vi "ConvertPB_LongDelay.vi"(0 "PB VLIW Array in":T2(array[cluster]) {"Output Bits" format="%x"}, 1 "Definitions":T1={"External MemorySize"=32768, "Internal Memory Size"=512, "Overhead Ticks"=3, "Min Delay Loops"=3, "Loop Count Correction"=1, "Long Delay Loop Count Correction"=2, "Min Instruction Ticks"=6, "Long Delay Ticks"=4294967295, "Clock Period (s)"=1e-08, "Overhead Time (s)"=3e-08, "Min Instruction Cycle Time (s)"=9e-08, "Long Delay Time (s) "=42.94967298} {"Long Delay Time (s)" format="%.8p"; "Min Instruction Cycle Time (s)" format="%.0p"; "Overhead Time (s)" format="%.0p"; "Clock Period (s)" format="%.0p"; "Long Delay Ticks" format="%.0x"}, 2 "error in (no error)":errorcluster, 3 "Full trigger mask":u32 format="%x") -> (5 "PB VLIW Array out":T2(array[cluster]) {"Output Bits" format="%x"}, 6 "error out":errorcluster)   [LabVIEW 2013, in "PulseBlaster.lvlib"]
doc: "Accounts for the strange clocking in of the line following a trigger while the PB is waiting for an external analog trigger."
uses:
  PulseBlaster.lvlib
panel:
  in  "BeginLoop pointer":u32
  # "(Period*Long D Ticks)+Overhead time"
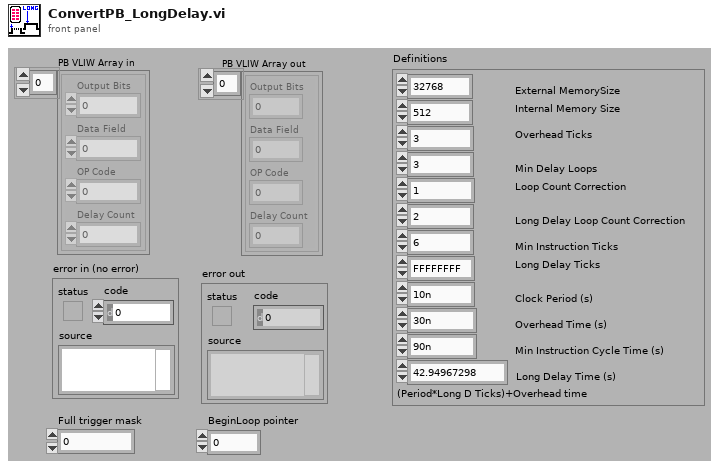
[diagram p1: front panel]
types:
  T1 = cluster{"External MemorySize":u16, "Internal Memory Size":u16, "Overhead Ticks":u8, "Min Delay Loops":u8, "Loop Count Correction":u8, "Long Delay Loop Count Correction":u8, "Min Instruction Ticks":u8, "Long Delay Ticks":u64, "Clock Period (s)":dbl, "Overhead Time (s)":dbl, "Min Instruction Cycle Time (s)":dbl, "Long Delay Time (s) ":dbl}
  T2 = cluster{"Output Bits":u32, "Data Field":u32, "OP Code":u8, "Delay Count":u64}[]
  T3 = cluster{"Output Bits":u32, "Data Field":u32, "OP Code":u8, "Delay Count":u32}[]
  T4 = cluster{"Output Bits":u32, "Data Field":u32, "OP Code":u8, u32}
  T5 = cluster{"Output Bits":u32, "Data Field":u32, "OP Code":u8, "Delay Count":u64}
  T6 = cluster{"Output Bits":u32, "BeginLoop pointer":u32, "OP Code":u8, "Delay Count":u64}
  T7 = cluster{"Output Bits":u32, "BeginLoop pointer":u32, "OP Code":u8, "Delay Count":u64}[]
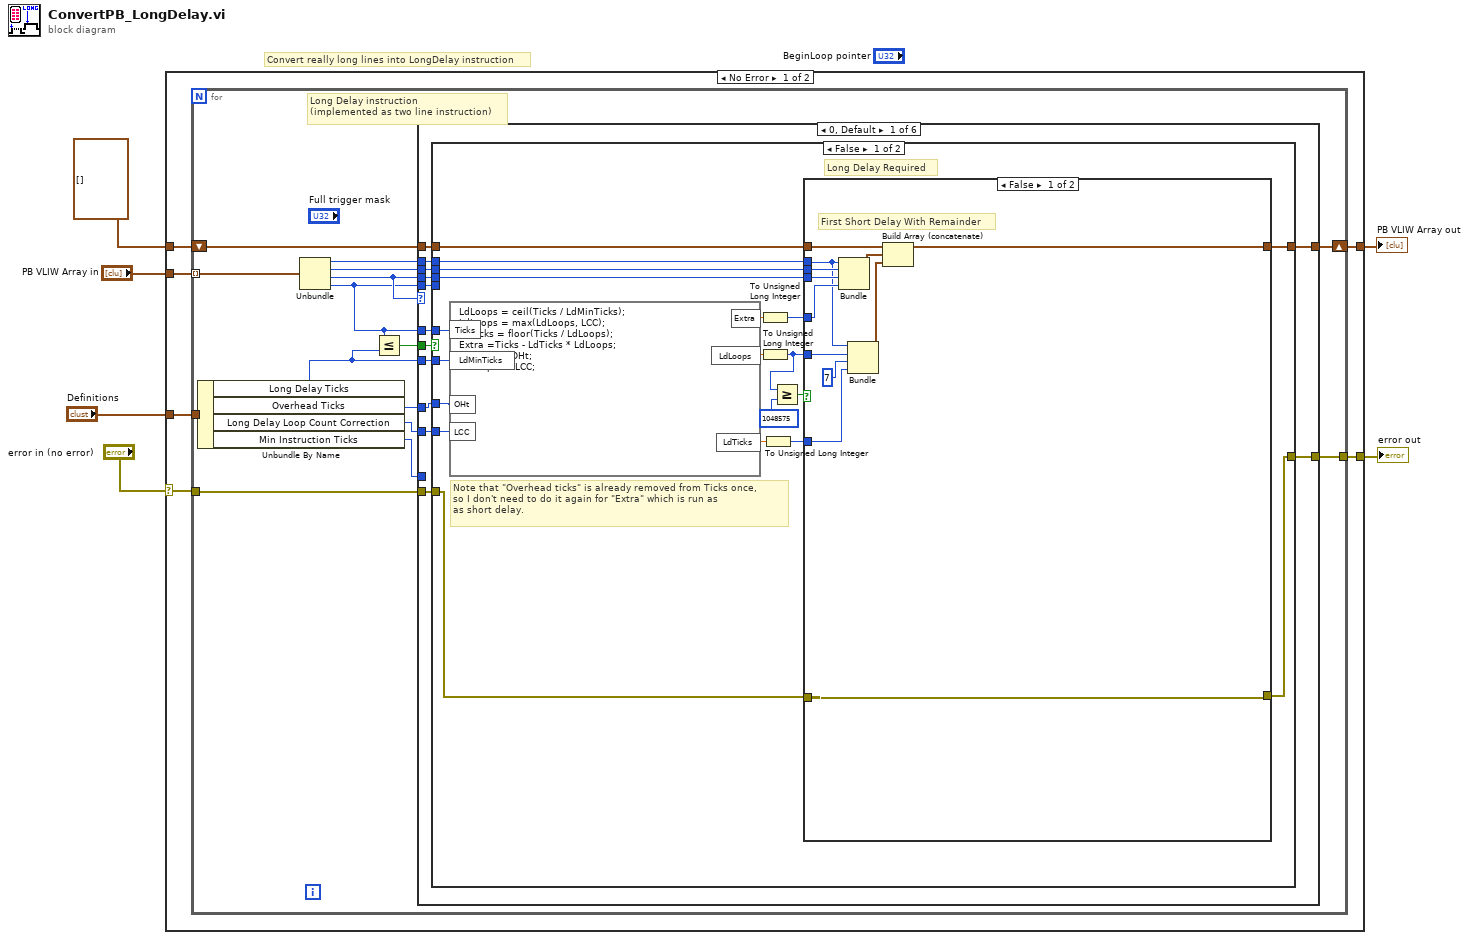
[diagram p0: block diagram]
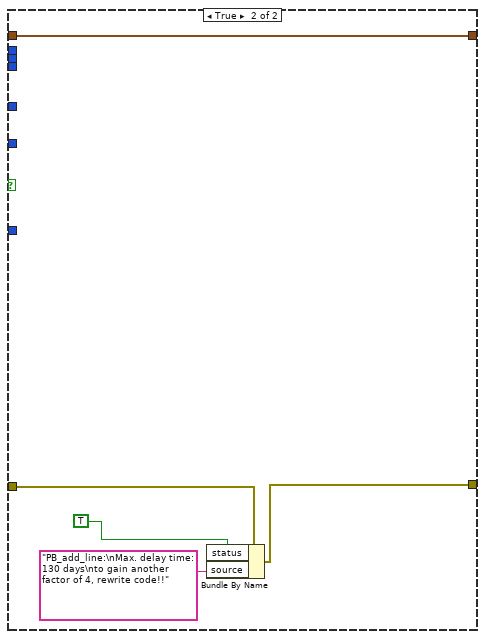
[diagram p2: hidden frame]
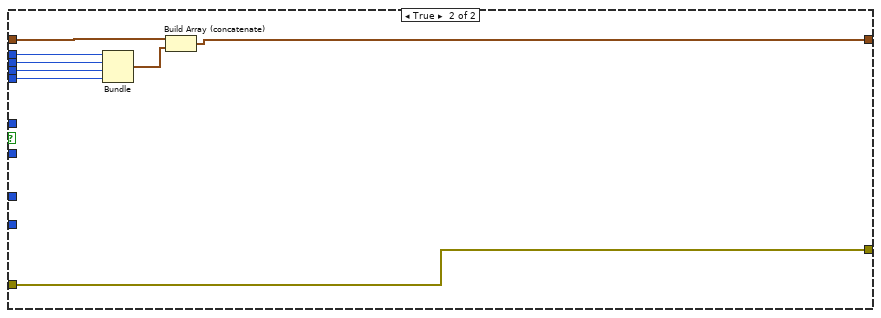
[diagram p3: hidden frame]
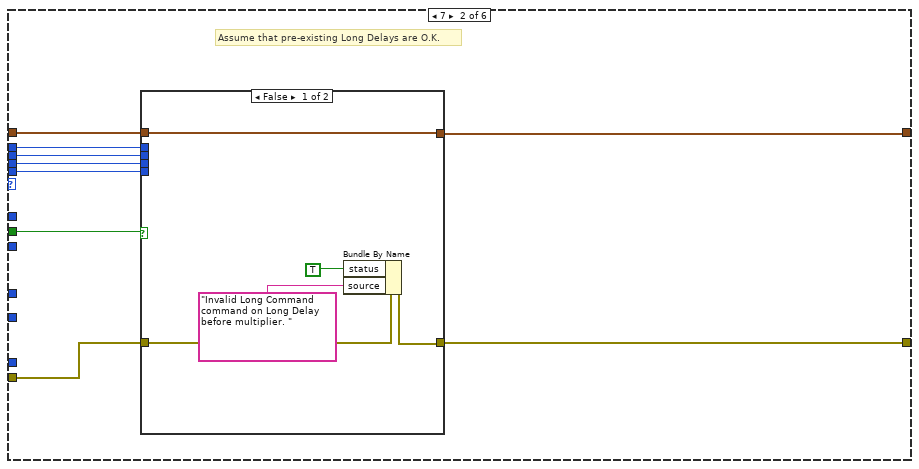
[diagram p4: hidden frame]
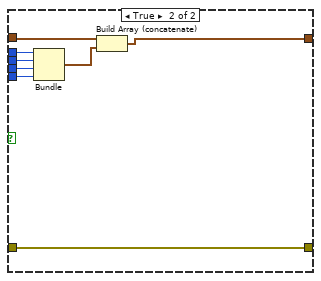
[diagram p5: hidden frame]
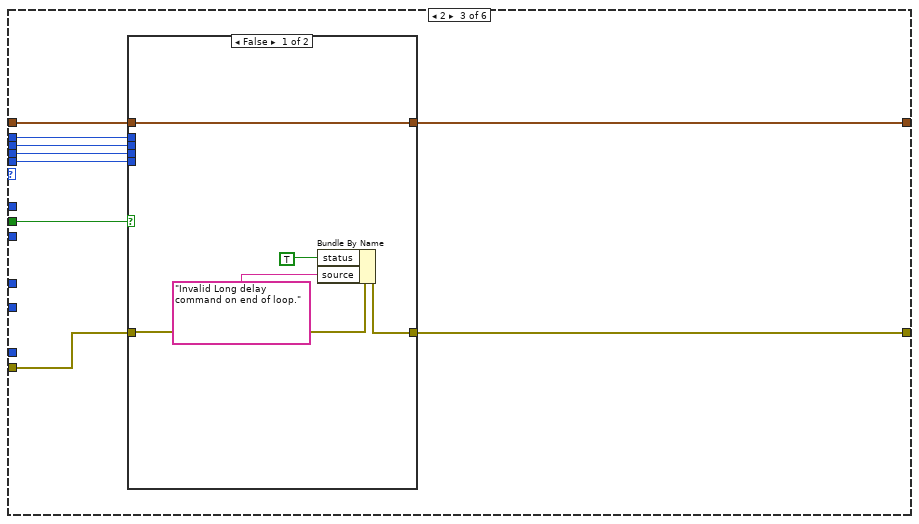
[diagram p6: hidden frame]
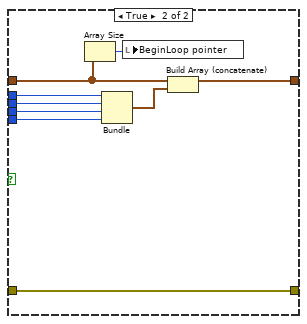
[diagram p7: hidden frame]
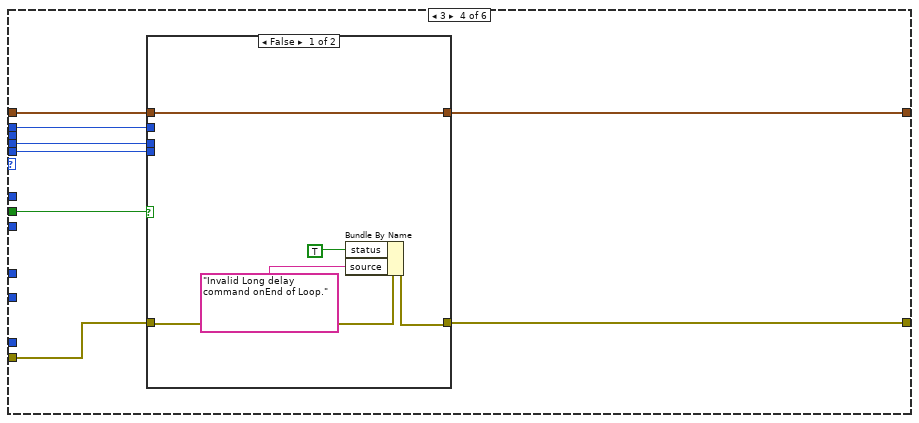
[diagram p8: hidden frame]
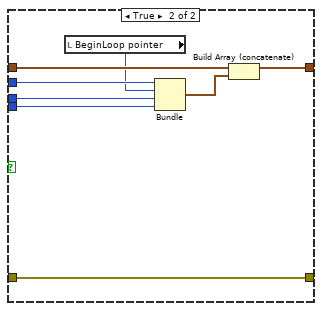
[diagram p9: hidden frame]
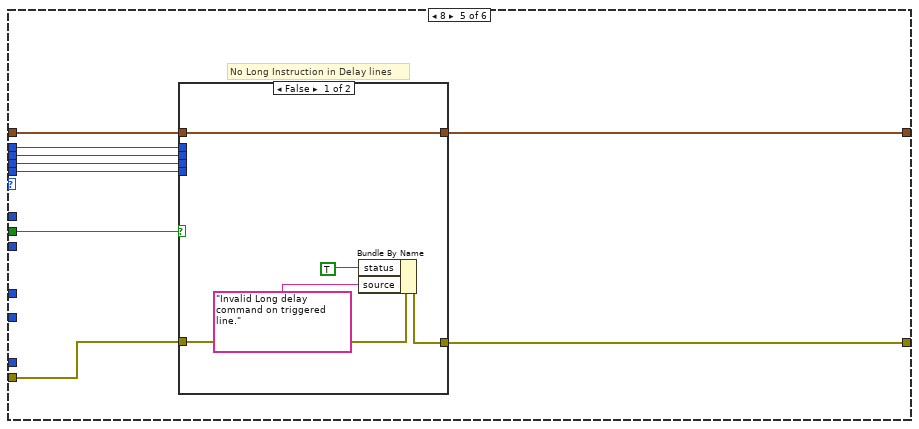
[diagram p10: hidden frame]
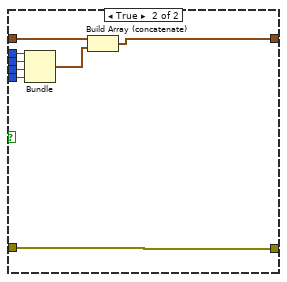
[diagram p11: hidden frame]
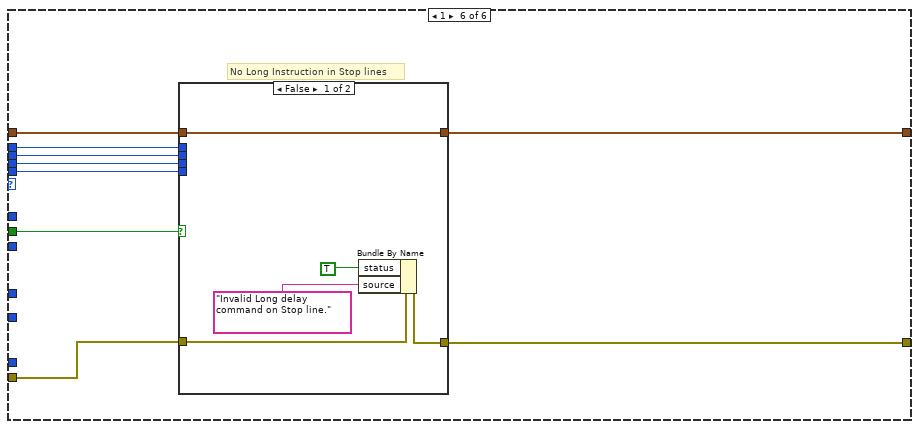
[diagram p12: hidden frame]
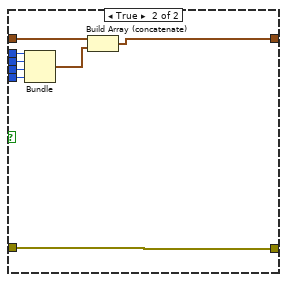
[diagram p13: hidden frame]
diagram:
  # "Convert really long lines into LongDelay instruction"
  n1 = case shown="No Error" "error in (no error)" {
    selector: "error in (no error)" -> [w8 w195]
    tunnel: T3 [] -> [w12 _]
    tunnel: [w11 w196] -> w5
    tunnel: "PB VLIW Array in" -> [w10 w196]
    tunnel: [w9 w195] -> w3
    tunnel: "Definitions" -> [w7 _]
    frame No Error {
      n2 = for {
        tunnel: w10 -> [w27] mode=indexing
        shift-right: [w22] -> w11
        shift-left: w12 -> [w25]
        tunnel: w8 -> [w24]
        tunnel: [w23] -> w9
        tunnel: w7 -> [w17]
        # "Long Delay instruction \n(implemented as two line instruction)"
        n3 = Unbundle By Name(w17) -> ("Long Delay Ticks"=w13:u64, "Overhead Ticks"=w14:u8, "Long Delay Loop Count Correction"=w15:u8, "Min Instruction Ticks"=w16:u8)
        n4 = Unbundle(w27) -> ("Output Bits"=w20:u32, "Data Field"=w26:u32, "OP Code"=w21:u8, "Delay Count"=w18:u64)
        n5 = Less Or Equal?(x=w18, y=w13) -> (x <= y?=w19:bool)
        n6 = case shown="0, Default" w21 {
          tunnel: w26 -> [w34 w87 w115 _ w153 w175]
          tunnel: w21 -> [w33 w86 w114 w137 w152 w174]
          tunnel: w18 -> [w32 w85 w113 w136 w151 w173]
          tunnel: w25 -> [w40 w93 w110 w135 w159 w181]
          tunnel: w24 -> [w37 w91 w109 w132 w158 w180]
          tunnel: [w36 w90 w108 w131 w157 w179] -> w23
          tunnel: w14 -> [w29 _ _ _ _ _]
          tunnel: w16 -> [_ _ _ _ _ _]
          tunnel: w20 -> [w35 w88 w112 w134 w154 w176]
          tunnel: [w39 w92 w111 w133 w156 w178] -> w22
          tunnel: w19 -> [w38 w89 w107 w130 w155 w177]
          tunnel: w18 -> [w31 _ _ _ _ _]
          tunnel: w13 -> [w30 _ _ _ _ _]
          tunnel: w15 -> [w28 _ _ _ _ _]
          frame 0, Default {
            n7 = case shown="False" w38 {
              tunnel: w40 -> [w55 w82]
              tunnel: [w54 w81] -> w39
              tunnel: w37 -> [w57 w84]
              tunnel: [w56 w84] -> w36
              tunnel: w35 -> [w50 w80]
              tunnel: w34 -> [w49 w79]
              tunnel: w33 -> [w48 w78]
              tunnel: w32 -> [_ w77]
              tunnel: w31 -> [w58 _]
              tunnel: w30 -> [w59 _]
              tunnel: w29 -> [w42 _]
              tunnel: w28 -> [w41 _]
              frame False {
                # "Note that \"Overhead ticks\" is already removed from Ticks once,\nso I don't need to do it again for \"Extra\" which is run as \nas short delay."
                # "Long Delay Required"
                n8 = formula code="LdLoops = ceil(Ticks / LdMinTicks);\nLdLoops = max(LdLoops, LCC);\nLdTicks = floor(Ticks / LdLoops);\nExtra =Ticks - LdTicks * LdLoops;\nLdTicks -= OHt;\nLdLoops -= LCC;"("LdMinTicks"=w59, "Ticks"=w58, "OHt"=w42, "LCC"=w41) -> ("LdLoops"=w44:dbl, "LdTicks"=w46:dbl, "Extra"=w51:dbl)
                n9 = To Unsigned Long Integer(number=w51) -> (unsigned 32bit integer=w47:u32)
                n10 = To Unsigned Long Integer(number=w44) -> (unsigned 32bit integer=w43:u32)
                n11 = To Unsigned Long Integer(number=w46) -> (unsigned 32bit integer=w45:u32)
                n12 = Greater Or Equal?(x=w43, y=1048575) -> (x >= y?=w53:bool)
                n13 = case shown="False" w53 {
                  tunnel: w57 -> [w71 w74]
                  tunnel: [w71 w73] -> w56
                  tunnel: w55 -> [w67 w72]
                  tunnel: [w65 w72] -> w54
                  tunnel: w47 -> [w66 _]
                  tunnel: w50 -> [w63 _]
                  tunnel: w49 -> [w70 _]
                  tunnel: w48 -> [w69 _]
                  tunnel: w45 -> [w61 _]
                  tunnel: w43 -> [w62 _]
                  frame False {
                    # "First Short Delay With Remainder"
                    n14 = Bundle("Output Bits"=w63, "Data Field"=w70, "OP Code"=w69, w66) -> (w68:T4)  [unwired: 1 out]
                    n15 = Bundle("Output Bits"=w63, w62, u8 7, w61) -> (w60:cluster{"Output Bits":u32, u32, u8, u32})  [unwired: 1 out]
                    n16 = Build Array (concatenate)(w67, w68, w60) -> (w65:T2)
                  }
                  frame True {
                    n17 = Bundle By Name(cluster=w74, "status"=TRUE, "source"="PB_add_line:\nMax. delay time: 130 days\nto gain another factor of 4, rewrite code!!") -> (w73:errorcluster)
                  }
                }
              }
              frame True {
                n18 = Bundle("Output Bits"=w80, "Data Field"=w79, "OP Code"=w78, "Delay Count"=w77) -> (w83:T5)  [unwired: 1 out]
                n19 = Build Array (concatenate)(w82, w83) -> (w81:T2)
              }
            }
          }
          frame 7 {
            # "Assume that pre-existing Long Delays are O.K."
            n20 = case shown="False" w89 {
              tunnel: w93 -> [w98 w104]
              tunnel: [w98 w103] -> w92
              tunnel: w91 -> [w95 w106]
              tunnel: [w94 w106] -> w90
              tunnel: w88 -> [_ w102]
              tunnel: w87 -> [_ w101]
              tunnel: w86 -> [_ w100]
              tunnel: w85 -> [_ w99]
              frame False {
                n21 = Bundle By Name(cluster=w95, "status"=TRUE, "source"="Invalid Long Command  command on Long Delay before multiplier. ") -> (w94:errorcluster)
              }
              frame True {
                n22 = Bundle("Output Bits"=w102, "Data Field"=w101, "OP Code"=w100, "Delay Count"=w99) -> (w105:T5)  [unwired: 1 out]
                n23 = Build Array (concatenate)(w104, w105) -> (w103:T2)
              }
            }
          }
          frame 2 {
            n24 = case shown="False" w107 {
              tunnel: w115 -> [_ w129]
              tunnel: w114 -> [_ w128]
              tunnel: w113 -> [_ w127]
              tunnel: w112 -> [_ w126]
              tunnel: [w116 w125] -> w111
              tunnel: w110 -> [w116 w122]
              tunnel: w109 -> [w118 w121]
              tunnel: [w117 w121] -> w108
              frame False {
                n25 = Bundle By Name(cluster=w118, "status"=TRUE, "source"="Invalid Long delay command on end of loop.") -> (w117:errorcluster)
              }
              frame True {
                n26 = Array Size(array=w122) -> (size(s)=w123:i32)
                n27 = Bundle("Output Bits"=w126, "Data Field"=w129, "OP Code"=w128, "Delay Count"=w127) -> (w124:T5)  [unwired: 1 out]
                n28 = local write "BeginLoop pointer"(w123) -> ()
                n29 = Build Array (concatenate)(w122, w124) -> (w125:T2)
              }
            }
          }
          frame 3 {
            n30 = case shown="False" w130 {
              tunnel: w137 -> [_ w150]
              tunnel: w136 -> [_ w149]
              tunnel: w135 -> [w138 w148]
              tunnel: w134 -> [_ w147]
              tunnel: [w138 w146] -> w133
              tunnel: w132 -> [w140 w143]
              tunnel: [w139 w143] -> w131
              frame False {
                n31 = Bundle By Name(cluster=w140, "status"=TRUE, "source"="Invalid Long delay command onEnd of Loop.") -> (w139:errorcluster)
              }
              frame True {
                n32 = local read "BeginLoop pointer"() -> (w144:u32)
                n33 = Bundle("Output Bits"=w147, "BeginLoop pointer"=w144, "OP Code"=w150, "Delay Count"=w149) -> (w145:T6)  [unwired: 1 out]
                n34 = Build Array (concatenate)(w148, w145) -> (w146:T7)
              }
            }
          }
          frame 8 {
            # "No Long Instruction in Delay lines"
            n35 = case shown="False" w155 {
              tunnel: w159 -> [w160 w167]
              tunnel: w158 -> [w164 w172]
              tunnel: [w163 w172] -> w157
              tunnel: [w160 w166] -> w156
              tunnel: w154 -> [_ w171]
              tunnel: w153 -> [_ w170]
              tunnel: w152 -> [_ w169]
              tunnel: w151 -> [_ w168]
              frame False {
                n36 = Bundle By Name(cluster=w164, "status"=TRUE, "source"="Invalid Long delay command on triggered line.") -> (w163:errorcluster)
              }
              frame True {
                n37 = Bundle("Output Bits"=w171, "Data Field"=w170, "OP Code"=w169, "Delay Count"=w168) -> (w165:T5)  [unwired: 1 out]
                n38 = Build Array (concatenate)(w167, w165) -> (w166:T2)
              }
            }
          }
          frame 1 {
            # "No Long Instruction in Stop lines"
            n39 = case shown="False" w177 {
              tunnel: w181 -> [w182 w189]
              tunnel: w180 -> [w186 w194]
              tunnel: [w185 w194] -> w179
              tunnel: [w182 w188] -> w178
              tunnel: w176 -> [_ w193]
              tunnel: w175 -> [_ w192]
              tunnel: w174 -> [_ w191]
              tunnel: w173 -> [_ w190]
              frame False {
                n40 = Bundle By Name(cluster=w186, "status"=TRUE, "source"="Invalid Long delay command on Stop line.") -> (w185:errorcluster)
              }
              frame True {
                n41 = Bundle("Output Bits"=w193, "Data Field"=w192, "OP Code"=w191, "Delay Count"=w190) -> (w187:T5)  [unwired: 1 out]
                n42 = Build Array (concatenate)(w189, w187) -> (w188:T2)
              }
            }
          }
        }
      }
    }
    frame Error {
    }
  }
  "error out" <- w3
  "PB VLIW Array out" <- w5
